vi "KM101_StartCtrl.vi"(10 "reference in":refnum<k7>) -> (2 "reference out":refnum<k7>)   [LabVIEW 2018, in "KIM101lib.lvlib"]
uses:
  KIM101lib.lvlib
  <vilib>/Utility/error.llb/DialogType.ctl
panel:
  out "lVoltage":i32
  out "lStepRate":i32
  out "lStepAccn":i32
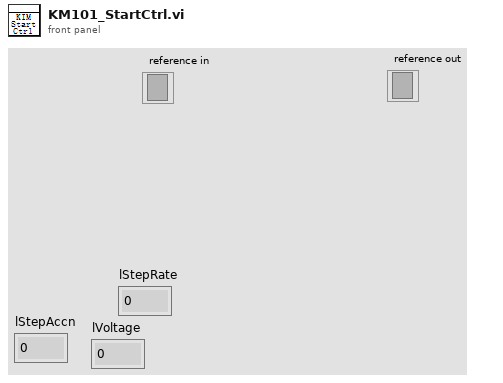
[diagram p1: front panel]
types:
  T1 = typedef "DialogType.ctl" = u16
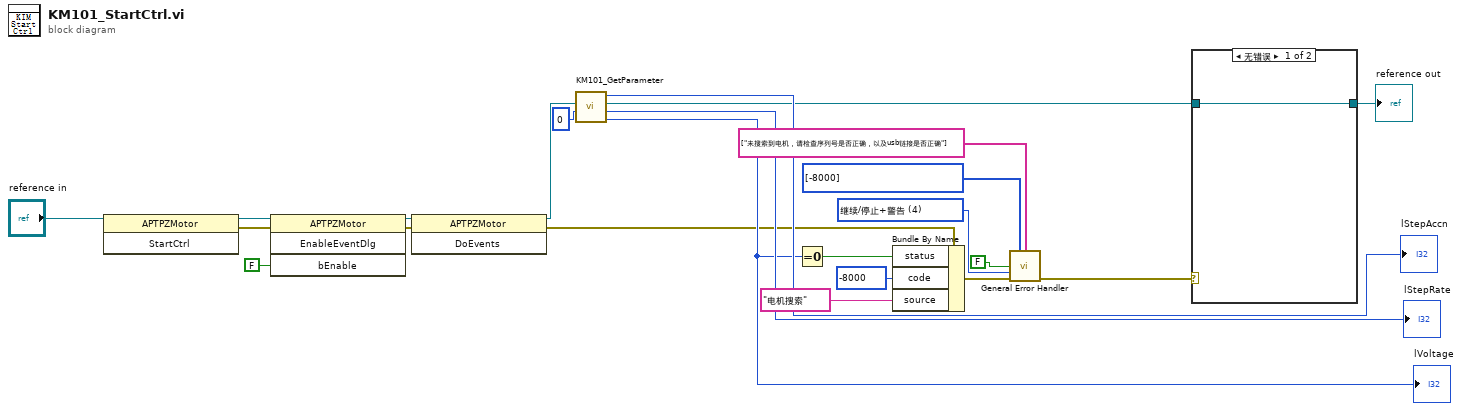
[diagram p0: block diagram]
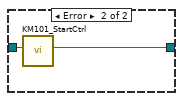
[diagram p2: hidden frame]
diagram:
  w19 = T1 4 items=["无对话框", "确定信息", "继续或停止信息", "确定信息＋警告", "继续/停止+警告"] ("type of dialog (OK msg:1)")
  n1 = invoke class="APTPZMotor" method="StartCtrl"(reference="reference in") -> (reference out=w22:refnum<k7>, error out=w7:errorcluster)  [unwired: 2 in, 1 out]
  n2 = invoke class="APTPZMotor" method="EnableEventDlg"(reference=w22, error in=w7, "bEnable"=FALSE) -> (reference out=w20:refnum<k7>, error out=w6:errorcluster)  [unwired: 1 in, 2 out]
  n3 = invoke class="APTPZMotor" method="DoEvents"(reference=w20, error in=w6) -> (reference out=w8:refnum<k7>, error out=w5:errorcluster)  [unwired: 1 in, 1 out]
  n4 = call "KM101_GetParameter.vi"("Channel"=0, "reference in"=w8) -> ("lVoltage"=w15:i32, "lStepRate"=→"lStepRate":i32, "reference out"=w4:refnum<k7>, "lStepAccn"=→"lStepAccn":i32)  [unwired: 6 in]
  "lVoltage" <- w15
  n5 = Equal To 0?(x=w15) -> (x = 0?=w14:bool)
  n6 = Bundle By Name(cluster=w5, "status"=w14, "code"=-8000, "source"="电机搜索" ("error source (\" \")")) -> (w2:errorcluster)
  n7 = call <vilib>:"General Error Handler.vi"("[user-defined codes]"=i32[] [-8000], "[user-defined descriptions]"=string[] ["未搜索到电机，请检查序列号是否正确，以及usb链接是否正确"], "search ni.com link visible?(T)"=FALSE, "type of dialog (OK msg:1)"=w19, "error in (no error)"=w2) -> ("error out"=w1:errorcluster)  [unwired: 6 in, 4 out]
  n8 = case shown="无错误" w1 {
    tunnel: w4 -> [w24 w26]
    tunnel: [w24 w25] -> w3
    frame No Error {
    }
    frame Error {
      n9 = call "KM101_StartCtrl.vi"("reference in"=w26) -> ("reference out"=w25:refnum<k7>)  [unwired: 10 in]
    }
  }
  "reference out" <- w3
